vi "Práctica_03.vi"() -> ()   [LabVIEW 2020]
panel:
  in  "Valor Mínimo":dbl=31.0
  in  "Valor Máximo":dbl=33.0 format="%#_13g"
  out "Actuador":bool
  out "Dato Actual":dbl
  out "Gráfica de Temperatura":dbl[](graph)
  out "Bandera":bool
  in  "stop":bool
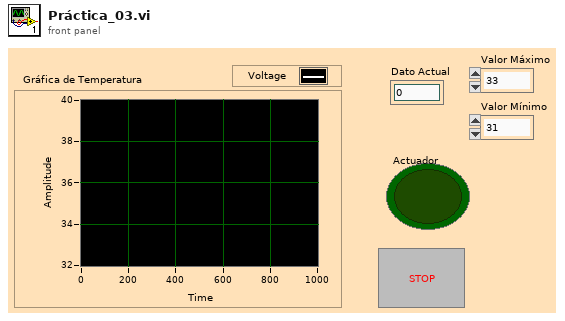
[diagram p1: front panel]
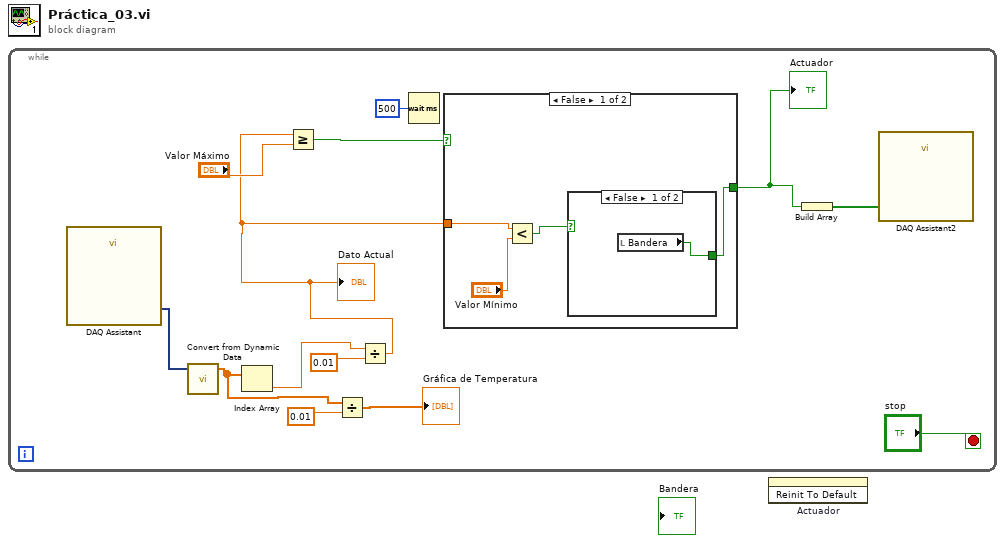
[diagram p0: block diagram]
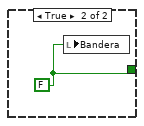
[diagram p2: hidden frame]
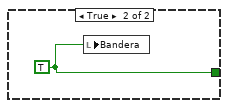
[diagram p3: hidden frame]
diagram:
  n1 = while {
    stop <- "stop" stop-if-true
    n2 = call "DAQ Assistant"() -> ("data"=w2:dynamicdata)  [unwired: 17 in, 2 out]
    n3 = call "Convert from Dynamic Data"("Dynamic Data Type"=w2) -> ("Array"=w7:dbl[])  [unwired: 3 in]
    n4 = Index Array(array=w7) -> (element=w5:dbl)  [unwired: 1 in]
    n5 = Divide(x=w7, y=0.01) -> (x/y=→"Gráfica de Temperatura":dbl[])
    n6 = Divide(x=w5, y=0.01) -> (x/y=w4:dbl)
    "Dato Actual" <- w4
    n7 = Greater Or Equal?(x=w4, y="Valor Máximo") -> (x >= y?=w8:bool)
    n8 = Wait (ms)(milliseconds to wait=u32 500) -> ()  [unwired: 1 out]
    n9 = case shown="False" w8 {
      tunnel: w4 -> [w17 _]
      tunnel: [w16 w20] -> w3
      frame False {
        n10 = Less?(x=w17, y="Valor Mínimo") -> (x < y?=w15:bool)
        n11 = case shown="False" w15 {
          tunnel: [w18 w19] -> w16
          frame False {
            n12 = local read "Bandera"() -> (w18:bool)
          }
          frame True {
            w19 = FALSE
            n13 = local write "Bandera"(w19) -> ()
          }
        }
      }
      frame True {
        w20 = TRUE
        n14 = local write "Bandera"(w20) -> ()
      }
    }
    "Actuador" <- w3
    n15 = Build Array(w3) -> (w1:bool[])
    n16 = call "DAQ Assistant2"("data"=w1) -> ()  [unwired: 17 in, 2 out]
  }
  n17 = invoke on="Actuador" class="Bool (strict)" method="Reinit To Default"() -> ()  [unwired: 3 in, 3 out]
